vi "Configure Auto Zero Mode [AZ].vi"(8 "error in (no error)":errorcluster, 10 "auto zero mode (Off)":i32(ring) items=["On"=1, "Off"=0, "Once"=2], 11 "CS++DMM in":refnum<class "CS++DMM.lvclass">) -> (0 "error out":errorcluster, 3 "CS++DMM out":refnum<class "CS++DMM.lvclass">)   [LabVIEW 2013, in "CS++DMM.lvlib" / "CS++DMM.lvclass"]
doc: "This VI configures the auto zero mode of the DMM.\n\nNote:\n\n(1) This VI is part of the IviDmmAutoZero [AZ] extension group."
uses:
  CS++DMM.lvclass
  Core/Classes/CS++ProcessVariables/ProcessVariable/PV.lvclass
  Core/Classes/CS++ProcessVariables/ProcessVariable/PV.lvclass/PV.ctl
  CS++DMM.lvclass/CS++DMM.ctl
  Core/Classes/CS++ProcessVariables/PVConnection/PVConnection.lvclass
  Core/Classes/CS++ProcessVariables/ProcessVariable/Write Data.vi
  Core/Classes/CS++ProcessVariables/ProcessVariable/Write Timestamp.vi
  Core/Classes/CS++ProcessVariables/ProcessVariable/Write Quality.vi
  Core/Classes/CS++ProcessVariables/ProcessVariable/Write status.vi
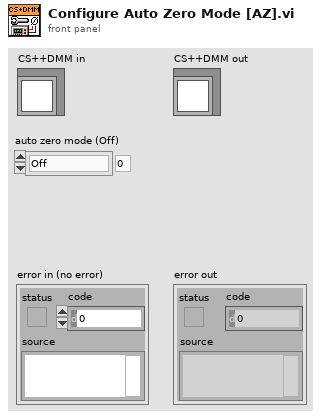
[diagram p1: front panel]
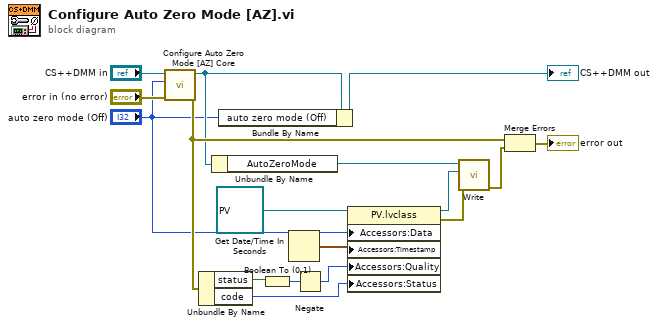
[diagram p0: block diagram]
diagram:
  n1 = call-dynamic "Configure Auto Zero Mode [AZ] Core.vi"("error in (no error)"="error in (no error)", "auto zero mode (Off)"="auto zero mode (Off)", "CS++DMM in"="CS++DMM in") -> ("error out"=w5:errorcluster, "CS++DMM out"=w3:refnum<class "CS++DMM.lvclass">)  [unwired: 7 in]
  n2 = Unbundle By Name(w5) -> ("status"=w14:bool, "code"=w11:i32)
  n3 = Unbundle By Name(w3) -> ("AutoZeroMode"=w7:refnum<class "PVConnection.lvclass">)
  n4 = Bundle By Name(cluster=w3, "auto zero mode (Off)"="auto zero mode (Off)") -> (→"CS++DMM out":refnum<class "CS++DMM.lvclass">)
  n5 = Boolean To (0,1)(Boolean=w14) -> (0, 1=w13:i16)
  n6 = Get Date/Time In Seconds() -> (seconds since 1Jan1904=w10:timestamp)
  n7 = Negate(x=w13) -> (-x=w12:i16)
  n8 = property class="PV.lvclass"(reference=refnum<class "PV.lvclass"> refnum ("CS++ProcessVariables.lvlib:PV.lvclass"), "Accessors:Data"="auto zero mode (Off)", "Accessors:Timestamp"=w10, "Accessors:Quality"=w12, "Accessors:Status"=w11) -> (reference out=w8:refnum<class "PV.lvclass">, error out=w9:errorcluster)  [unwired: 1 in]
  n9 = call-dynamic "Write.vi"("error in (no error)"=w9, "PV"=w8, "PVConnection in"=w7) -> ("error out"=w6:errorcluster)  [unwired: 7 in, 1 out]
  n10 = Merge Errors(w5, w6) -> (→"error out":errorcluster)
